vi "Get RemIO UI Ref.vi"(8 "error in (no error)":errorcluster, 11 "11115 in":refnum<class "11115.lvclass">) -> (0 "error out":errorcluster, 2 "VI Refnum":refnum<vi>, 3 "11115 out":refnum<class "11115.lvclass">)   [LabVIEW 2016, in "Modules.lvlib" / "11115.lvclass"]
uses:
  11115.lvclass
  11115 UI.vi
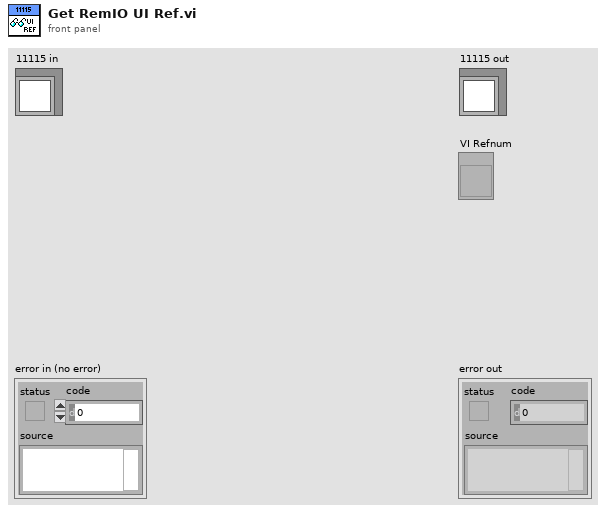
[diagram p1: front panel]
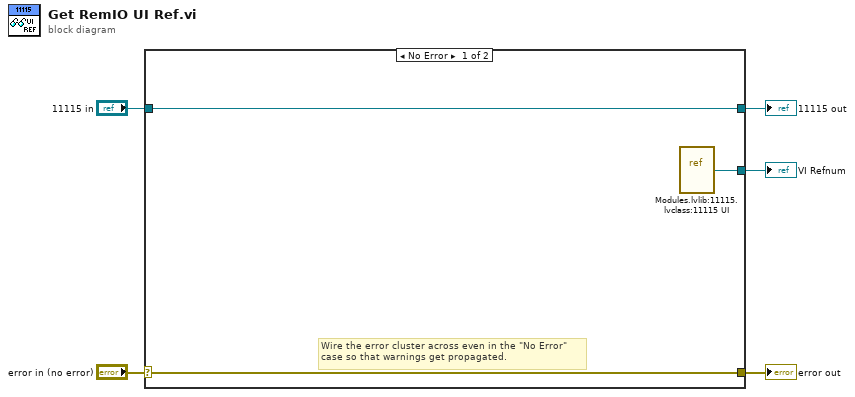
[diagram p0: block diagram]
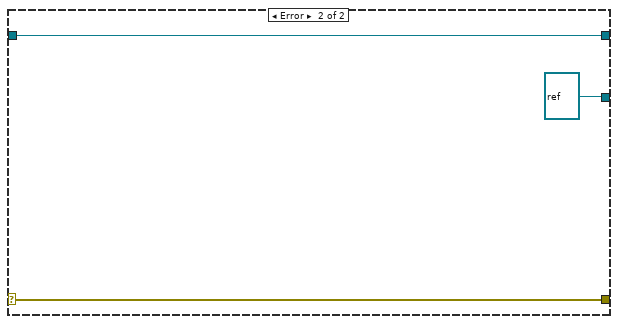
[diagram p2: hidden frame]
diagram:
  n1 = case shown="No Error" "error in (no error)" {
    selector: "error in (no error)" -> [w7 w11]
    tunnel: [w7 w11] -> w5
    tunnel: [w8 w10] -> w1
    tunnel: "11115 in" -> [w8 w10]
    tunnel: [w6 refnum<vi> refnum] -> w2
    frame No Error {
      # "Wire the error cluster across even in the \"No Error\"\ncase so that warnings get propagated."
      n2 = vi-ref "Modules.lvlib:11115.lvclass:11115 UI.vi"() -> (w6:refnum<vi>)
    }
    frame Error {
    }
  }
  "error out" <- w5
  "11115 out" <- w1
  "VI Refnum" <- w2
